vi "Tabor.vi"(7 "Init?":bool, 8 "error in (no error)":errorcluster, 11 "Tabor handle in":refnum<k15>) -> (0 "error out":errorcluster, 3 "Tabor handleout":refnum<k15>)   [LabVIEW 2022 SP3]
uses:
  Pulsers/PulserGlobals.vi
panel:
  in  "operation mode":i32(ring) items=["Continuous"=0, "Burst"=1, "Gated"=1001, "Triggered"=1002]
  in  "Trigger Source":T1={"source"=1, "trigger slope"=2003, "trigger level"=1.6} {"trigger level" format="%.2p"; "trigger slope" items=["Positive"=2003, "Negative"=2002]; "source" items=["External"=1, "Internal"=3, "Software Trigger"=2]}
  in  "Burst Settings":T2={"Internal Rate (Hz)"=100.0, "Burst Count "=1} {"Burst Count" min=1 max=50000; "Internal Rate (Hz)" min=0.002 max=1000000.0 format="%.2f"}
  in  "Enable Output":bool
  in  "Exit Program":bool
  in  "Basic Wvfrm":T3={"waveform"=1, "Freq or Time"=1000.0, "Amplitude (Vpp)"=0.1, "Offset (V)"=0.0, "duty cycle"=50.0} {"duty cycle" format="%.2p"; "waveform" items=["Sine"=1, "Square"=2, "Triangle"=3, "Ramp Up"=4, "Ramp Down"=5, "DC"=6, "Ramp"=1001, "Pulse"=1005, "Sinc"=1002, "Gaussian"=1003, "Exponential"=1004, "Noise"=1006]; "Offset (V)" min=-10.0 max=10.0 format="%.2f"; "Amplitude (Vpp)" min=0.001 max=20.0 format="%.2f"; "Freq or Time" min=1e-06 max=80000000.0 format="%^#.2e"}
  # "Simple commands for Tabor control"
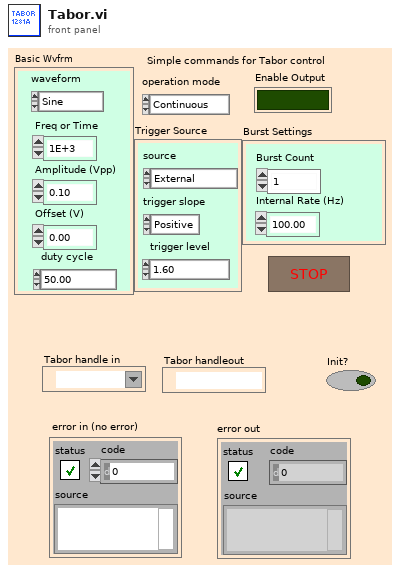
[diagram p1: front panel]
types:
  T1 = cluster{"source":i32, "trigger slope":i32, "trigger level":dbl}
  T2 = cluster{"Internal Rate (Hz)":dbl, "Burst Count ":i32}
  T3 = cluster{"waveform":i32, "Freq or Time":dbl, "Amplitude (Vpp)":dbl, "Offset (V)":dbl, "duty cycle":dbl}
  T4 = cluster{"Therapy frequency (MHz)":dbl, "Therapy amplitude (mV)":dbl, "time therapy on (s)":dbl, "Therapy Delay (ms) ":dbl, "Time (s)":dbl}
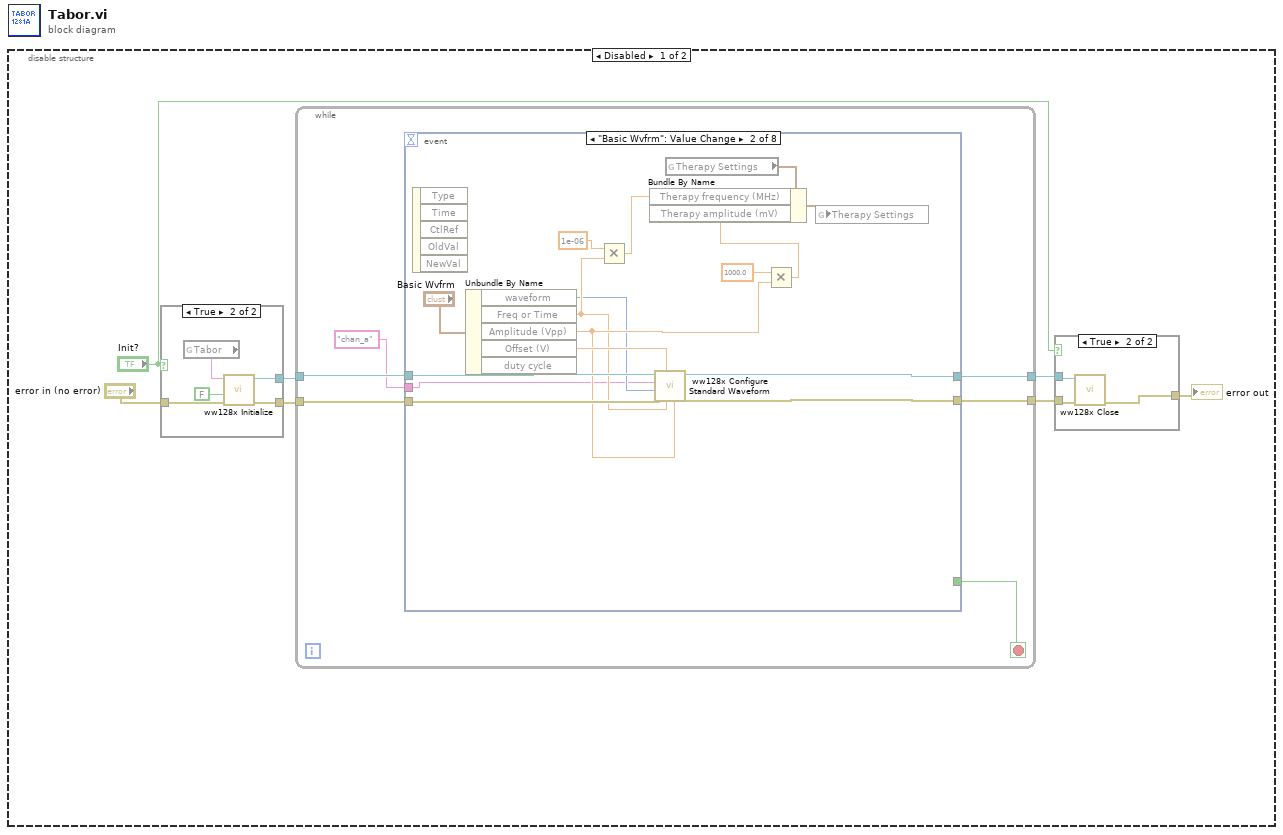
[diagram p0: block diagram]
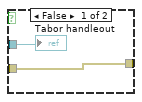
[diagram p2: hidden frame]
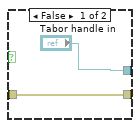
[diagram p3: hidden frame]
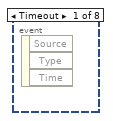
[diagram p4: hidden frame]
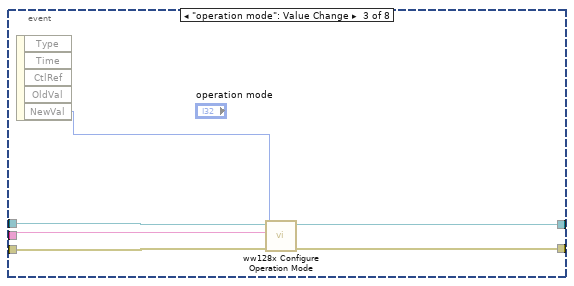
[diagram p5: hidden frame]
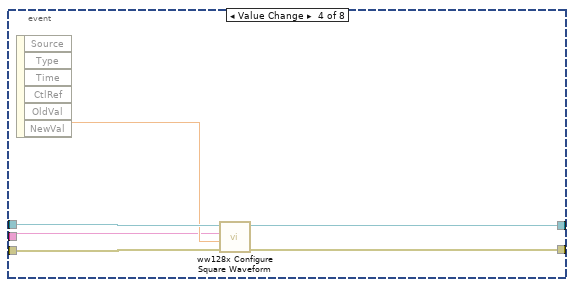
[diagram p6: hidden frame]
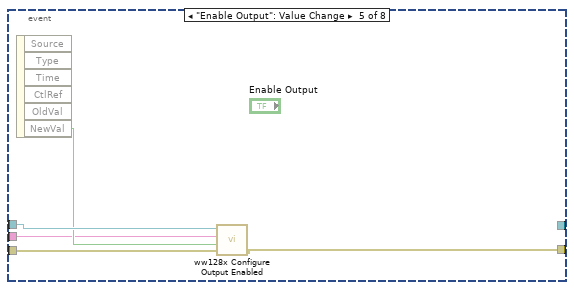
[diagram p7: hidden frame]
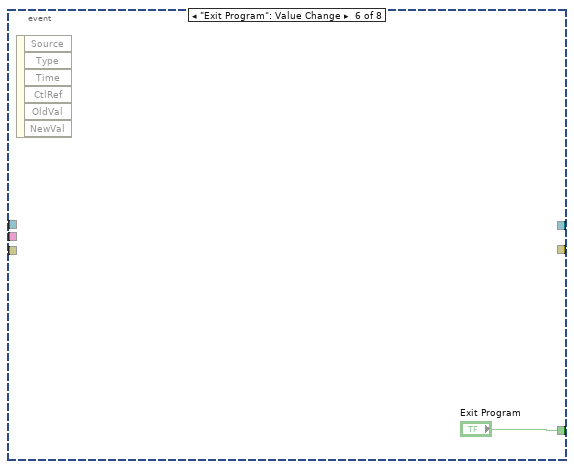
[diagram p8: hidden frame]
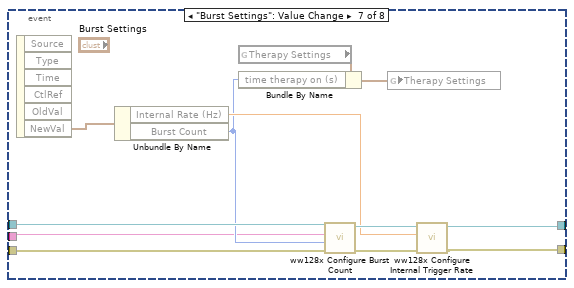
[diagram p9: hidden frame]
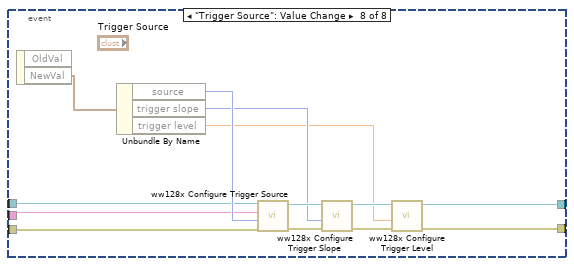
[diagram p10: hidden frame]
diagram:
  n1 = disable-structure shown="Disabled" {
    frame Disabled {
      n2 = case shown="True" "Init?" {
        tunnel: ["Tabor handle in" w19] -> w7
        tunnel: [w13 w18] -> w6
        tunnel: "error in (no error)" -> [w13 w17]
        frame False {
        }
        frame True {
          n3 = global read "PulserGlobals.vi" "Tabor"() -> (w15:string)
          n4 = call <instrlib>:"ww128x Initialize.vi"("error in (no error)"=w17, "reset device (Yes)"=FALSE ("Reset (T: Reset)"), "resource name"=w15) -> ("error out"=w18:errorcluster, "instrument handle out"=w19:refnum<k15>)  [unwired: 7 in]
        }
      }
      n5 = while {
        tunnel: w7 -> [w25]
        tunnel: w6 -> [w24]
        tunnel: [w23] -> w2
        tunnel: [w22] -> w4
        stop <- w21 stop-if-true
        n6 = event shown="[1] \"Basic Wvfrm\": Value Change" {
          selector: _ -> [_ _ _ _ _ _ _ _]
          dyn-events: _ -> [_ _ _ _ _ _ _ _]
          timeout: _ -> [_ _ _ _ _ _ _ _]
          tunnel: w25 -> [_ w40 w46 w51 w58 _ w69 w83]
          tunnel: w24 -> [_ w39 w45 w53 w57 _ w71 w82]
          tunnel: [_ w32 w43 w50 _ _ w68 w76] -> w23
          tunnel: [_ w31 w44 w52 w56 _ w70 w77] -> w22
          tunnel: [_ _ _ _ _ "Exit Program" _ _] -> w21
          tunnel: "chan_a" ("channel name (\"CHAN_A\")") -> [_ w26 w42 w48 w54 _ w60 w74]
          event Timeout {
            n7 = event-data() -> ()  [unwired: 4 out]
          }
          event "Basic Wvfrm": Value Change {
            n8 = event-data() -> ()  [unwired: 6 out]
            n9 = Unbundle By Name("Basic Wvfrm") -> ("waveform"=w33:i32, "Freq or Time"=w34:dbl, "Amplitude (Vpp)"=w35:dbl, "Offset (V)"=w36:dbl)  [unwired: 1 out]
            n10 = Multiply(x=1e-06, y=w34) -> (x*y=w27:dbl)
            n11 = call <instrlib>:"ww128x Configure Standard Waveform.vi"("amplitude"=w35, "frequency"=w34, "dc offset"=w36, "error in (no error)"=w39, "waveform"=w33, "channel name"=w26, "instrument handle"=w40) -> ("error out"=w31:errorcluster, "instrument handle out"=w32:refnum<k15>)  [unwired: 3 in]
            n12 = global read "PulserGlobals.vi" "Therapy Settings"() -> (w30:T4)
            n13 = Multiply(x=1000.0, y=w35) -> (x*y=w28:dbl)
            n14 = Bundle By Name(cluster=w30, "Therapy frequency (MHz)"=w27, "Therapy amplitude (mV)"=w28) -> (w29:T4)
            n15 = global write "PulserGlobals.vi" "Therapy Settings"(w29) -> ()
          }
          event "operation mode": Value Change {
            n16 = event-data() -> ("NewVal"=w47:i32)  [unwired: 5 out]
            n17 = call <instrlib>:"ww128x Configure Operation Mode.vi"("error in (no error)"=w45, "operation mode (Continuous)"=w47, "channel name (\"CHAN_A\")"=w42, "instrument handle"=w46) -> ("error out"=w44:errorcluster, "instrument handle out"=w43:refnum<k15>)  [unwired: 6 in]
          }
          event "Basic Wvfrm.duty cycle": Value Change {
            n18 = event-data() -> ("NewVal"=w49:dbl)  [unwired: 6 out]
            n19 = call <instrlib>:"ww128x Configure Square Waveform.vi"("error in (no error)"=w53, "Duty Cycle (50)"=w49, "Channel Name (\"CHAN_A\")"=w48, "instrument handle"=w51) -> ("error out"=w52:errorcluster, "instrument handle out"=w50:refnum<k15>)  [unwired: 6 in]
          }
          event "Enable Output": Value Change {
            n20 = event-data() -> ("NewVal"=w55:bool)  [unwired: 6 out]
            n21 = call <instrlib>:"ww128x Configure Output Enabled.vi"("error in (no error)"=w57, "channel enabled (False)"=w55, "channel name (\"CHAN_A\")"=w54, "instrument handle"=w58) -> ("error out"=w56:errorcluster)  [unwired: 6 in, 1 out]
          }
          event "Exit Program": Value Change {
            n22 = event-data() -> ()  [unwired: 7 out]
          }
          event "Burst Settings": Value Change {
            n23 = event-data() -> ("NewVal"=w67:T2)  [unwired: 6 out]
            n24 = Unbundle By Name(w67) -> ("Internal Rate (Hz)"=w64:dbl, "Burst Count"=w61:i32)
            n25 = global read "PulserGlobals.vi" "Therapy Settings"() -> (w63:T4)
            n26 = Bundle By Name(cluster=w63, "time therapy on (s)"=w61) -> (w62:T4)
            n27 = call <instrlib>:"ww128x Configure Burst Count.vi"("error in (no error)"=w71, "burst count (2)"=w61, "channel name (\"CHAN_A\")"=w60, "instrument handle"=w69) -> ("error out"=w65:errorcluster, "instrument handle out"=w66:refnum<k15>)  [unwired: 6 in]
            n28 = global write "PulserGlobals.vi" "Therapy Settings"(w62) -> ()
            n29 = call <instrlib>:"ww128x Configure Internal Trigger Rate.vi"("error in (no error)"=w65, "trigger rate (1.0e-3)"=w64, "instrument handle"=w66) -> ("error out"=w70:errorcluster, "instrument handle out"=w68:refnum<k15>)  [unwired: 7 in]
          }
          event "Trigger Source": Value Change {
            n30 = event-data() -> ("NewVal"=w75:T1)  [unwired: 2 out]
            n31 = Unbundle By Name(w75) -> ("source"=w84:i32, "trigger slope"=w73:i32, "trigger level"=w72:dbl)
            n32 = call <instrlib>:"ww128x Configure Trigger Source.vi"("error in (no error)"=w82, "trigger source (External)"=w84, "channel name (\"CHAN_A\")"=w74, "instrument handle"=w83) -> ("error out"=w80:errorcluster, "instrument handle out"=w81:refnum<k15>)  [unwired: 6 in]
            n33 = call <instrlib>:"ww128x Configure Trigger Slope.vi"("error in (no error)"=w80, "Trigger Slope (Positive)"=w73, "instrument handle"=w81) -> ("error out"=w79:errorcluster, "instrument handle out"=w78:refnum<k15>)  [unwired: 7 in]
            n34 = call <instrlib>:"ww128x Configure Trigger Level.vi"("error in (no error)"=w79, "Trigger Level (1.6)"=w72, "instrument handle"=w78) -> ("error out"=w77:errorcluster, "instrument handle out"=w76:refnum<k15>)  [unwired: 7 in]
          }
        }
      }
      n35 = case shown="True" "Init?" {
        tunnel: w4 -> [w8 w12]
        tunnel: [w8 w11] -> w3
        tunnel: w2 -> [w9 w10]
        frame False {
          "Tabor handleout" <- w9
        }
        frame True {
          n36 = call <instrlib>:"ww128x Close.vi"("error in (no error)"=w12, "instrument handle"=w10) -> ("error out"=w11:errorcluster)  [unwired: 9 in]
        }
      }
      "error out" <- w3
    }
    frame Enabled {
    }
  }
